vi "lolazo.vi"() -> ()   [LabVIEW 2015]
panel:
  out "Cuadrado":dbl
  in  "Numeric":dbl
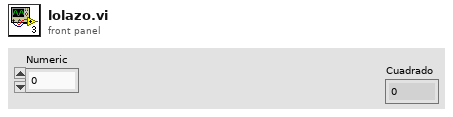
[diagram p1: front panel]
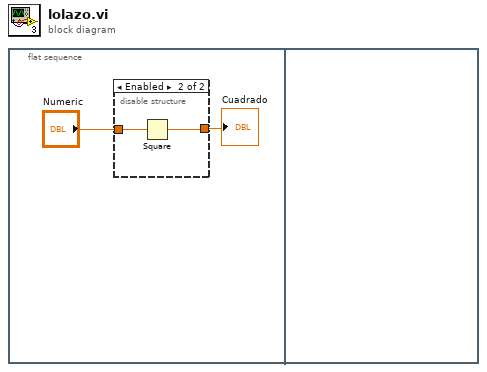
[diagram p0: block diagram]
diagram:
  n1 = flat-sequence {
    frame #0 {
      n2 = disable-structure shown="Enabled" {
        disable-tunnel: "Numeric" -> [_ w4]
        disable-tunnel: [_ w3] -> w1
        frame Disabled {
        }
        frame Enabled {
          n3 = Square(x=w4) -> (x^2=w3:dbl)
        }
      }
      "Cuadrado" <- w1
    }
    frame #1 {
    }
  }
